vi "startThread.vi"(0 "HGF_ThreadPool_Reference":refnum<class "HGF_Reference.lvclass">, 3 "timeout in ms (-1)":i32=-1, 5 "error in (no error)":errorcluster) -> (14 "dup HGF_ThreadPool_Reference":refnum<class "HGF_Reference.lvclass">, 17 "got object?":bool, 19 "error out":errorcluster)   [LabVIEW 2014, in "HGF_BaseClasses.lvlib" / "HGF_ThreadPool.lvclass"]
doc: "Start new threads."
uses:
  HGF_ThreadPool.lvclass
  HGF_ThreadWorker/HGF_ThreadWorker.lvclass
  HGF_Reference/HGF_Reference.lvclass
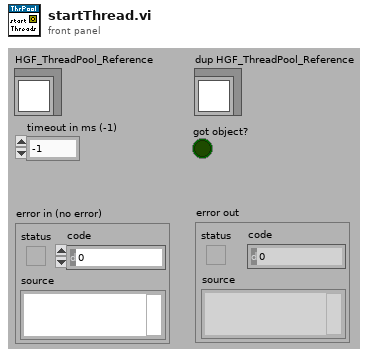
[diagram p1: front panel]
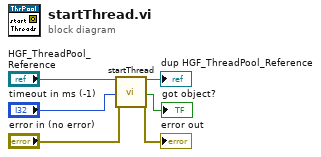
[diagram p0: block diagram]
diagram:
  n1 = call "startThread.vi"("HGF_ThreadPool_Reference"="HGF_ThreadPool_Reference", "timeout in ms (-1)"="timeout in ms (-1)", "error in (no error)"="error in (no error)") -> ("HGF_ThreadPool_Reference"=→"dup HGF_ThreadPool_Reference":refnum<class "HGF_Reference.lvclass">, "got object?"=→"got object?":bool, "error out"=→"error out":errorcluster)  [unwired: 2 in, 12 out]
